vi "MarginLeft.vi"(1 "输入":dbl[][](array[numeric])) -> (0 "输出":dbl)   [LabVIEW 2016]
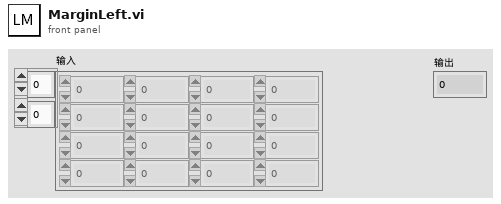
[diagram p1: front panel]
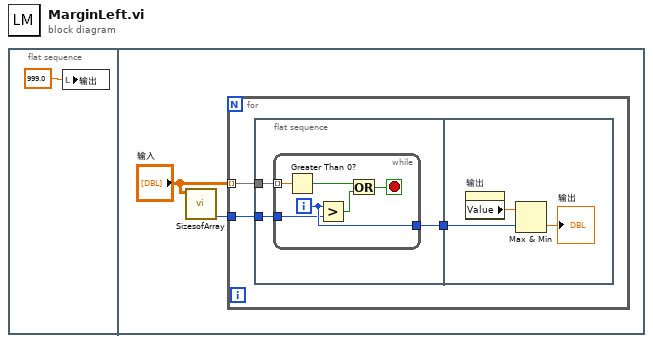
[diagram p0: block diagram]
diagram:
  n1 = flat-sequence {
    frame #0 {
      n2 = local write "输出"(999.0) -> ()
    }
    frame #1 {
      n3 = call "SizesofArray.vi"("数组"="输入") -> ("NumCols_r"=w2:i32)  [unwired: 7 in, 3 out]
      n4 = for {
        tunnel: "输入" -> [w6] mode=indexing
        tunnel: w2 -> [w4]
        n5 = flat-sequence {
          tunnel: w6 -> [w9]
          tunnel: [w8] -> w5
          tunnel: w4 -> [w7]
          tunnel: w5 -> [w17]
          frame #0 {
            n6 = while {
              tunnel: w9 -> [w15] mode=indexing
              tunnel: [w14] -> w8
              tunnel: w7 -> [w10]
              i -> [w14]
              stop <- w11 stop-if-true
              n7 = Greater Than 0?(x=w15) -> (x > 0?=w13:bool)
              n8 = Greater?(x=w14, y=w10) -> (0:w12:bool)
              n9 = Or(x=w13, y=w12) -> (x .or. y?=w11:bool)
            }
          }
          frame #1 {
            n10 = property on="输出" class="DigNum (严格)"() -> ("Value"=w18:dbl)  [unwired: 2 in, 2 out]
            n11 = Max & Min(x=w18, y=w17) -> (min(x,y)=→"输出":dbl)  [unwired: 1 out]
          }
        }
      }
    }
  }
